vi "saveToCSV.vi"() -> ()   [LabVIEW 2018]
uses:
  <vilib>/Utility/file.llb/Write Delimited Spreadsheet (string).vi
  <vilib>/Utility/file.llb/Write Delimited Spreadsheet (DBL).vi
panel:
  out "appended array":dbl[][](array[numeric])
  in  "file path (dialog if empty)":path
  in  "stop":bool
  out "Array":string[](array[string])
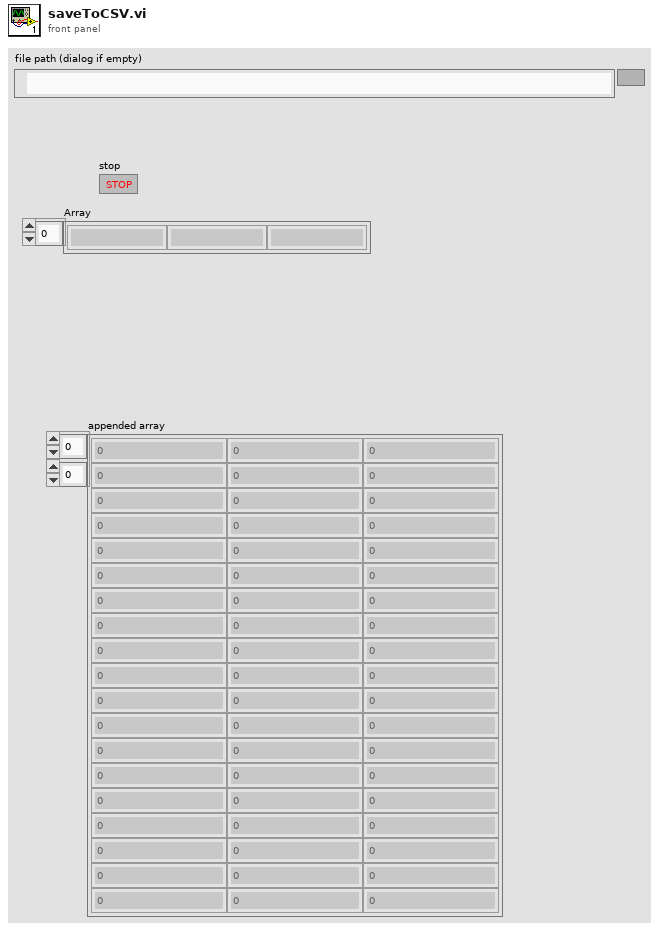
[diagram p1: front panel]
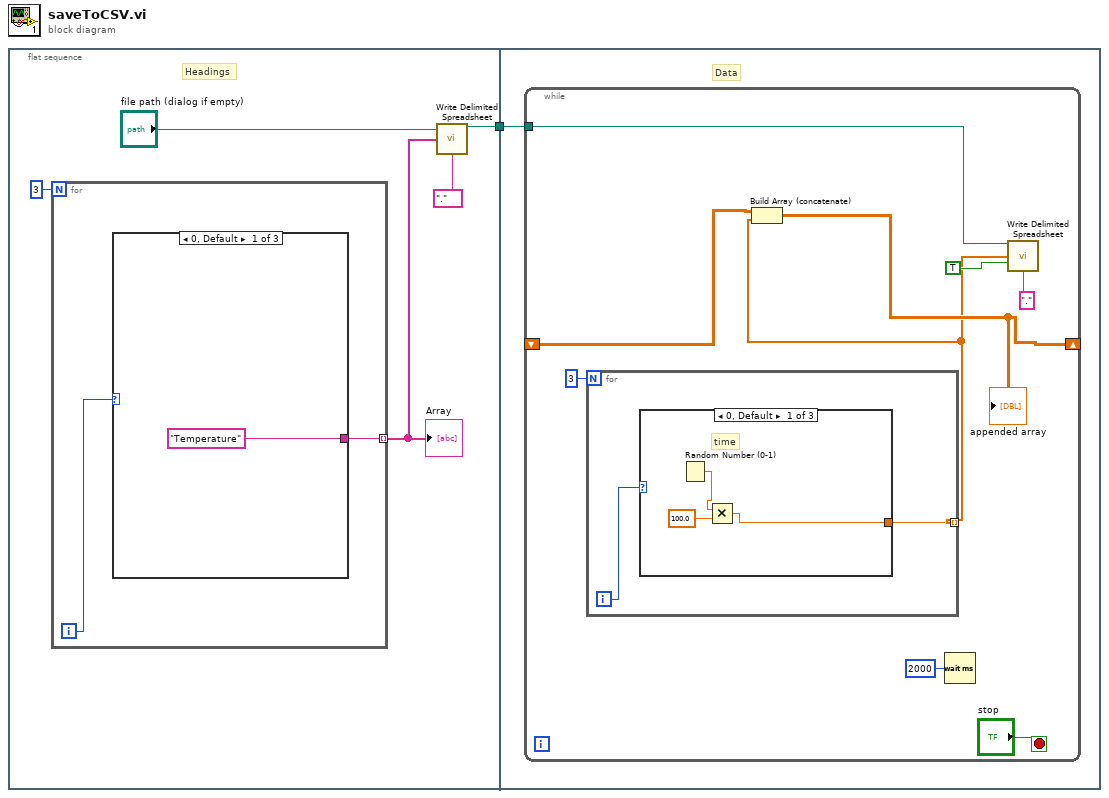
[diagram p0: block diagram]
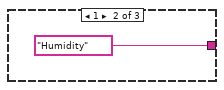
[diagram p2: hidden frame]
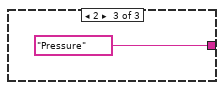
[diagram p3: hidden frame]
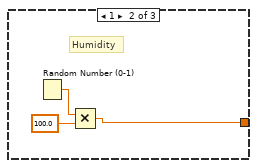
[diagram p4: hidden frame]
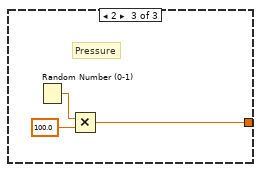
[diagram p5: hidden frame]
diagram:
  n1 = flat-sequence {
    tunnel: [w2] -> w1
    tunnel: w1 -> [w12]
    frame #0 {
      # "Headings"
      n2 = for {
        N: 3 -> [_]
        tunnel: [w7] -> w4 mode=indexing
        i -> [w8]
        n3 = case shown="0, Default" w8 {
          tunnel: ["Temperature" "Humidity" "Pressure"] -> w7
          frame 0, Default {
          }
          frame 1 {
          }
          frame 2 {
          }
        }
      }
      "Array" <- w4
      n4 = call-poly <vilib>:"Write Delimited Spreadsheet.vi"("file path (dialog if empty)"="file path (dialog if empty)", "1D data"=w4, "delimiter (\\t)"="." ("delimiter (\\t)")) -> ("new file path (Not A Path if cancelled)"=w2:path)  [unwired: 11 in, 1 out]
    }
    frame #1 {
      # "Data"
      n5 = while {
        tunnel: w12 -> [w19]
        shift-right: [w14] -> _
        shift-left: _ -> [w15]
        stop <- "stop" stop-if-true
        n6 = for {
          N: 3 -> [_]
          tunnel: [w22] -> w13 mode=indexing
          i -> [w23]
          n7 = case shown="0, Default" w23 {
            tunnel: [w24 w27 w30] -> w22
            frame 0, Default {
              # "time"
              n8 = Random Number (0-1)() -> (number: 0 to 1=w25:dbl)
              n9 = Multiply(x=w25, y=100.0) -> (x*y=w24:dbl)
            }
            frame 1 {
              # "Humidity"
              n10 = Random Number (0-1)() -> (number: 0 to 1=w28:dbl)
              n11 = Multiply(x=w28, y=100.0) -> (x*y=w27:dbl)
            }
            frame 2 {
              # "Pressure"
              n12 = Random Number (0-1)() -> (number: 0 to 1=w31:dbl)
              n13 = Multiply(x=w31, y=100.0) -> (x*y=w30:dbl)
            }
          }
        }
        n14 = Build Array (concatenate)(w15, w13) -> (w14:dbl[][])
        "appended array" <- w14
        n15 = Wait (ms)(milliseconds to wait=u32 2000) -> ()  [unwired: 1 out]
        n16 = call-poly <vilib>:"Write Delimited Spreadsheet.vi"("file path (dialog if empty)"=w19, "1D data"=w13, "append to file? (new file:F)"=TRUE, "delimiter (\\t)"="." ("delimiter (\\t)")) -> ()  [unwired: 10 in, 2 out]
      }
    }
  }
